vi "Create Stack Info.vi"(6 "Raw File Params":cluster{"raw offset":u32, "raw frame gap":u32}, 7 "nFrames":i32, 8 "error in (no error)":errorcluster, 10 "Camera Type":T3, 11 "Active Cameras":T1[](array[typedef])) -> (0 "error out":errorcluster, 2 "Stack Info":T2)   [LabVIEW 2023]
uses:
  Type Defs/Camera Type.ctl
  Type Defs/Stack Info.ctl
  Type Defs/Physical Camera Assignment.ctl
  <vilib>/Utility/error.llb/Trim Whitespace One-Sided.vi
  GLOBAL/GLOBAL Experiment Metadata.vi
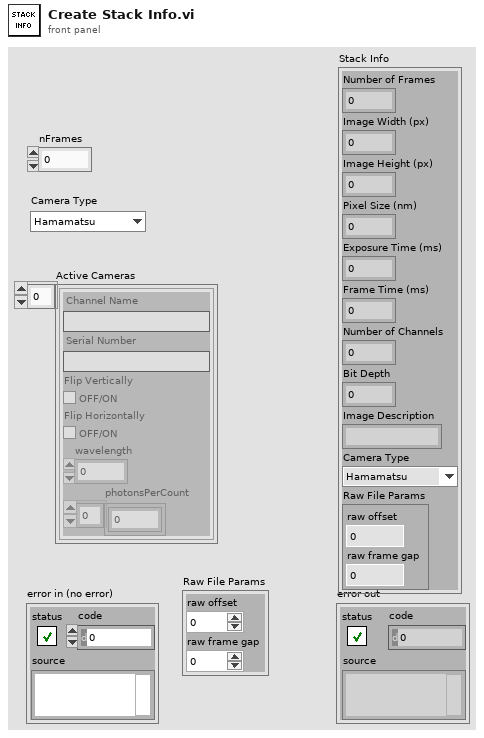
[diagram p1: front panel]
types:
  T1 = typedef "Physical Camera Assignment.ctl" = cluster{"Channel Name":string, "Serial Number":string, "Flip Vertically":bool, "Flip Horizontally":bool, "wavelength":i16, "photonsPerCount":dbl[]}
  T2 = typedef "Stack Info.ctl" = cluster{"Number of Frames":u32, "Image Width (px)":u32, "Image Height (px)":u32, "Pixel Size (nm)":dbl, "Exposure Time (ms)":dbl, "Frame Time (ms)":dbl, "Number of Channels":u32, "Bit Depth":u32, "Image Description":string, "Camera Type":T3, "Raw File Params":cluster{"raw offset":i32, "raw frame gap":i32}}
  T3 = typedef "Camera Type.ctl" = enum16{"Hamamatsu", "Andor", "Photometrics"}
  T4 = typedef "Camera Settings.ctl" = cluster{"Exposure Time (ms)":dbl, "Binning":enum16{"1x1", "2x2", "4x4"}, "Scan Mode":i32, "Frames to Acquire":dbl, "Pixel Correction":bool, "Frames to Skip":u32, "File Path":path, "Duty cycle":dbl, "ALEX":bool, "Shutter Enable":bool[], "fluidics trigger, ms (0=disabled)":dbl, "Bit Depth":u16, "Image Width (px)":u16, "Image Height (px)":u16, "Horizontal Offset (px)":u16, "Vertical Offset (px)":u16}
  T5 = cluster{"Shutter Enable":bool[], "Duty Cycle":dbl, "Wavelengths":dbl[], "ALEX?":bool}
  T6 = typedef "Stage Position.ctl" = cluster{"X (mm)":dbl, "Y (mm)":dbl, "Z (mm)":dbl}
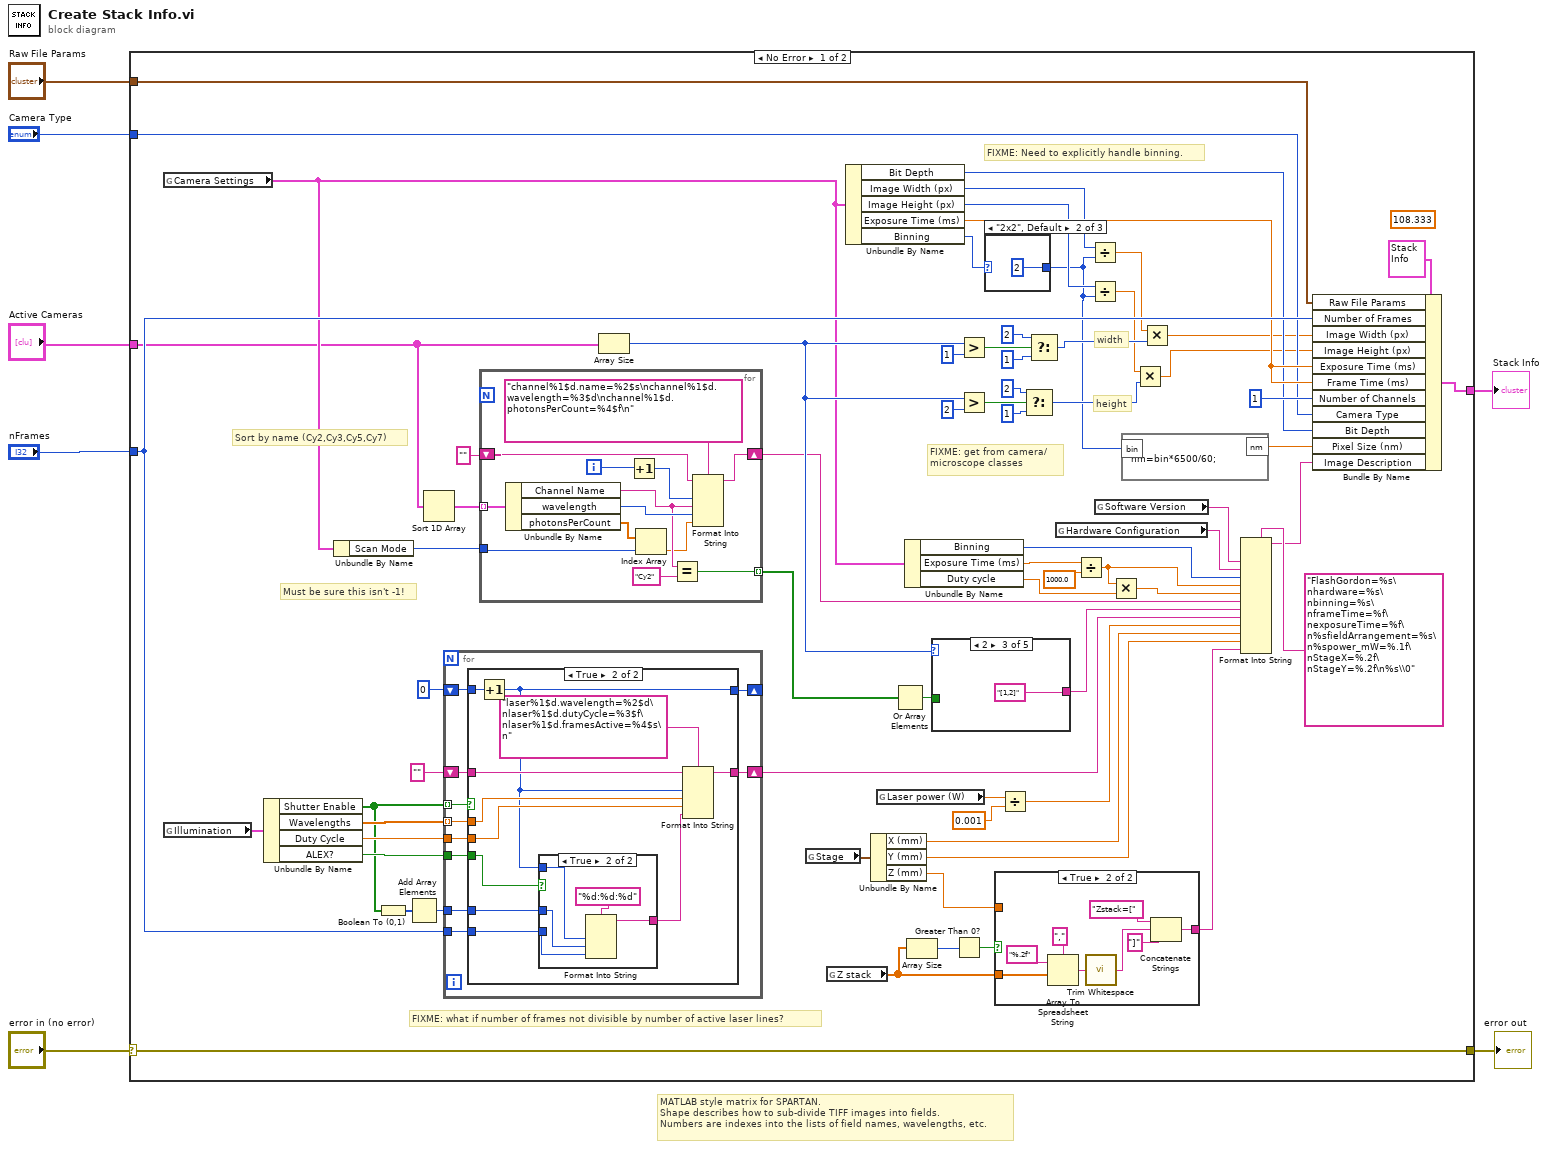
[diagram p0: block diagram]
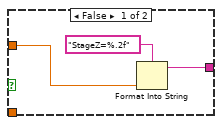
[diagram p2: hidden frame]
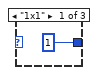
[diagram p3: hidden frame]
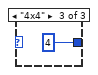
[diagram p4: hidden frame]
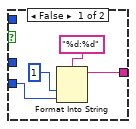
[diagram p6: hidden frame]
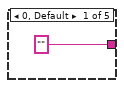
[diagram p7: hidden frame]
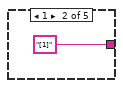
[diagram p8: hidden frame]
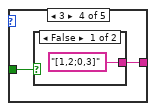
[diagram p9: hidden frame]
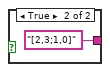
[diagram p10: hidden frame]
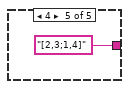
[diagram p11: hidden frame]
diagram:
  # "MATLAB style matrix for SPARTAN.\nShape describes how to sub-divide TIFF images into fields.\nNumbers are indexes into the lists of field names, wavelengths, etc."
  n1 = case shown="No Error" "error in (no error)" {
    selector: "error in (no error)" -> [w76 w144]
    tunnel: [w76 w144] -> w6
    tunnel: "nFrames" -> [w49 _]
    tunnel: [w66 _] -> w3
    tunnel: "Camera Type" -> [w34 _]
    tunnel: "Active Cameras" -> [w17 _]
    tunnel: "Raw File Params" -> [w8 _]
    frame No Error {
      (unwired) 108.333 ("Pixel Size (nm)")
      # "FIXME: get from camera/\nmicroscope classes"
      # "height"
      # "width"
      # "Must be sure this isn't -1!"
      # "FIXME: Need to explicitly handle binning."
      # "FIXME: what if number of frames not divisible by number of active laser lines?"
      # "Sort by name (Cy2,Cy3,Cy5,Cy7)"
      n2 = global read "GLOBAL Experiment Metadata.vi" "Camera Settings"() -> (w32:T4)
      n3 = global read "GLOBAL Experiment Metadata.vi" "Illumination"() -> (w58:T5)
      n4 = Unbundle By Name(w58) -> ("Shutter Enable"=w48:bool[], "Wavelengths"=w56:dbl[], "Duty Cycle"=w57:dbl, "ALEX?"=w55:bool)
      n5 = Unbundle By Name(w32) -> ("Scan Mode"=w31:i32)
      n6 = Boolean To (0,1)(Boolean=w48) -> (0, 1=w47:i16[])
      n7 = Add Array Elements(numeric array=w47) -> (sum=w46:i16)
      n8 = Sort 1D Array(array=w17) -> (sorted array=w63:T1[])
      n9 = for {
        tunnel: w48 -> [w100] mode=indexing
        tunnel: w57 -> [w96]
        tunnel: w56 -> [w97] mode=indexing
        tunnel: w55 -> [w95]
        shift-right: [w98] -> w53
        shift-left: "" -> [w99]
        shift-right: [w93] -> _
        shift-left: 0 -> [w94]
        tunnel: w49 -> [w92]
        tunnel: w46 -> [w91]
        n10 = case shown="True" w100 {
          tunnel: w99 -> [w102 w111]
          tunnel: [w102 w112] -> w98
          tunnel: w97 -> [_ w110]
          tunnel: w96 -> [_ w109]
          tunnel: w95 -> [_ w107]
          tunnel: [w101 w106] -> w93
          tunnel: w94 -> [w101 w108]
          tunnel: w92 -> [_ w105]
          tunnel: w91 -> [_ w103]
          frame False {
            # "ignore inactive laser line"
          }
          frame True {
            n11 = Increment(x=w108) -> (x+1=w106:i32)
            n12 = case shown="True" w107 {
              tunnel: w106 -> [_ w118]
              tunnel: w105 -> [w115 w120]
              tunnel: [w116 w122] -> w104
              tunnel: w103 -> [_ w119]
              frame False {
                n13 = Format Into String(format string="%d:%d", 1 ("input 1"), w115) -> (resulting string=w116:string)  [unwired: 2 in, 1 out]
              }
              frame True {
                n14 = Format Into String(format string="%d:%d:%d", w118, w119, w120) -> (resulting string=w122:string)  [unwired: 2 in, 1 out]
              }
            }
            n15 = Format Into String(format string="laser%1$d.wavelength=%2$d\nlaser%1$d.dutyCycle=%3$f\nlaser%1$d.framesActive=%4$s\n", initial string=w111, w106, w110, w109, w104) -> (resulting string=w112:string)  [unwired: 1 in, 1 out]
          }
        }
      }
      n16 = for {
        tunnel: w63 -> [w143] mode=indexing
        shift-right: [w140] -> w43
        shift-left: "" -> [w139]
        tunnel: [w136] -> w64 mode=indexing
        tunnel: w31 -> [w131]
        i -> [w135]
        # "Write spectral channel information (for now one channel per camera)"
        n17 = Unbundle By Name(w143) -> ("Channel Name"=w137:string, "wavelength"=w142:i16, "photonsPerCount"=w133:dbl[])
        n18 = Increment(x=w135) -> (x+1=w134:i32)
        n19 = Index Array(array=w133, index=w131) -> (element=w132:dbl)
        n20 = Equal?(x=w137, y="Cy2" ("x")) -> (x = y?=w136:bool)
        n21 = Format Into String(format string="channel%1$d.name=%2$s\nchannel%1$d.wavelength=%3$d\nchannel%1$d.photonsPerCount=%4$f\n", initial string=w139, w134, w137, w142, w132) -> (resulting string=w140:string)  [unwired: 1 in, 1 out]
      }
      n22 = Array Size(array=w17) -> (size(s)=w45:i32)
      n23 = global read "GLOBAL Experiment Metadata.vi" "Stage"() -> (w39:T6)
      n24 = global read "GLOBAL Experiment Metadata.vi" "Z stack"() -> (w16:dbl[])
      n25 = Unbundle By Name(w32) -> ("Bit Depth"=w33:u16, "Image Width (px)"=w29:u16, "Image Height (px)"=w28:u16, "Exposure Time (ms)"=w44:dbl, "Binning"=w30:enum16{"1x1", "2x2", "4x4"})
      n26 = Unbundle By Name(w39) -> ("X (mm)"=w11:dbl, "Y (mm)"=w10:dbl, "Z (mm)"=w12:dbl)
      n27 = global read "GLOBAL Experiment Metadata.vi" "Laser power (W)"() -> (w37:dbl)
      n28 = Or Array Elements(Boolean array=w64) -> (logical OR=w65:bool)
      n29 = Unbundle By Name(w32) -> ("Binning"=w51:enum16{"1x1", "2x2", "4x4"}, "Exposure Time (ms)"=w40:dbl, "Duty cycle"=w42:dbl)
      n30 = Array Size(array=w16) -> (size(s)=w14:i32)
      n31 = case shown="2" w45 {
        tunnel: w65 -> [_ _ _ w127 _]
        tunnel: ["" "[1]" "[1,2]" w126 "[2,3;1,4]"] -> w59
        frame 0, Default {
        }
        frame 1 {
        }
        frame 2 {
        }
        frame 3 {
          n32 = case shown="False" w127 {
            tunnel: ["[1,2;0,3]" "[2,3;1,0]"] -> w126
            frame False {
            }
            frame True {
            }
          }
        }
        frame 4 {
        }
      }
      n33 = Greater Than 0?(x=w14) -> (x > 0?=w15:bool)
      n34 = Greater?(x=w45, y=1) -> (0:w75:bool)
      n35 = Greater?(x=w45, y=2) -> (0:w74:bool)
      n36 = case shown="\"2x2\", Default" w30 {
        tunnel: [u16 1 ("Value in") u16 2 ("Value in") u16 4 ("Value in")] -> w18
        frame "1x1" {
        }
        frame "2x2", Default {
        }
        frame "4x4" {
        }
      }
      n37 = case shown="True" w15 {
        tunnel: w16 -> [_ w87]
        tunnel: [w78 w82] -> w9
        tunnel: w12 -> [w79 _]
        frame False {
          n38 = Format Into String(format string="StageZ=%.2f", w79) -> (resulting string=w78:string)  [unwired: 2 in, 1 out]
        }
        frame True {
          n39 = Array To Spreadsheet String(delimiter (Tab)=",", array=w87, 3:"%.2f" ("format string")) -> (spreadsheet string=w81:string)
          n40 = call <vilib>:"Trim Whitespace.vi"("string"=w81) -> ("trimmed string"=w80:string)  [unwired: 1 in]
          n41 = Concatenate Strings("Zstack=[" ("string"), w80, "]" ("string")) -> (w82:string)
        }
      }
      n42 = Divide(x=w37, y=0.001) -> (x/y=w13:dbl)
      n43 = Select(t=u16 2 ("f"), s=w74, f=u16 1) -> (s? t:f=w21:u16)
      n44 = Select(t=u16 2, s=w75, f=u16 1) -> (s? t:f=w25:u16)
      n45 = global read "GLOBAL Experiment Metadata.vi" "Hardware Configuration"() -> (w50:string)
      n46 = Divide(x=w40, y=1000.0) -> (x/y=w36:dbl)
      n47 = Divide(x=w29, y=w18) -> (x/y=w26:dbl)
      n48 = Divide(x=w28, y=w18) -> (x/y=w22:dbl)
      n49 = global read "GLOBAL Experiment Metadata.vi" "Software Version"() -> (w60:string)
      n50 = Multiply(x=w36, y=w42) -> (x*y=w41:dbl)
      n51 = formula code="nm=bin*6500/60;"("bin"=w18) -> ("nm"=w19:dbl)
      n52 = Multiply(x=w22, y=w21) -> (x*y=w23:dbl)
      n53 = Multiply(x=w26, y=w25) -> (x*y=w27:dbl)
      n54 = Format Into String(format string="FlashGordon=%s\nhardware=%s\nbinning=%s\nframeTime=%f\nexposureTime=%f\n%sfieldArrangement=%s\n%spower_mW=%.1f\nStageX=%.2f\nStageY=%.2f\n%s\\0" ("Image Description"), w60, w50, w51, w36, w41, w43, w59, w53, w13, w11, w10, w9) -> (resulting string=w20:string)  [unwired: 2 in, 1 out]
      n55 = Bundle By Name(cluster=T2 {"Number of Frames"=0, "Image Width (px)"=0, "Image Height (px)"=0, "Pixel Size (nm)"=0.0, "Exposure Time (ms)"=0.0, "Frame Time (ms)"=0.0, "Number of Channels"=0, "Bit Depth"=0, "Image Description"="", "Camera Type"=enum."Hamamatsu", "Raw File Params"={"raw offset"=0, "raw frame gap"=0}} ("Stack Info"), "Raw File Params"=w8, "Number of Frames"=w49, "Image Width (px)"=w27, "Image Height (px)"=w23, "Exposure Time (ms)"=w44, "Frame Time (ms)"=w44, "Number of Channels"=u32 1, "Camera Type"=w34, "Bit Depth"=w33, "Pixel Size (nm)"=w19, "Image Description"=w20) -> (w66:T2)
    }
    frame Error {
    }
  }
  "error out" <- w6
  "Stack Info" <- w3
